vi "Do Something Else and Wait for Reply.vi"(6 "wait for reply (T)":bool=TRUE, 8 "error in (no error)":errorcluster, 9 "X":dbl, 10 "Do Something Else Message":string, 11 "Module ID":i32=-1) -> (0 "error out":errorcluster, 1 "timed out?":bool, 2 "Reply Payload":T1)   [LabVIEW 2018, in "CE14 eMIC module.lvlib"]
doc: "Send the Do Something Else request to the Module's Main.vi.\n_____\nBased on DQMH Project Template 6.0.0.91."
uses:
  CE14 eMIC module.lvlib
  Do Something Else and Wait (Reply Payload)--cluster.ctl
  Do Something Else and Wait for Reply Argument--cluster.ctl
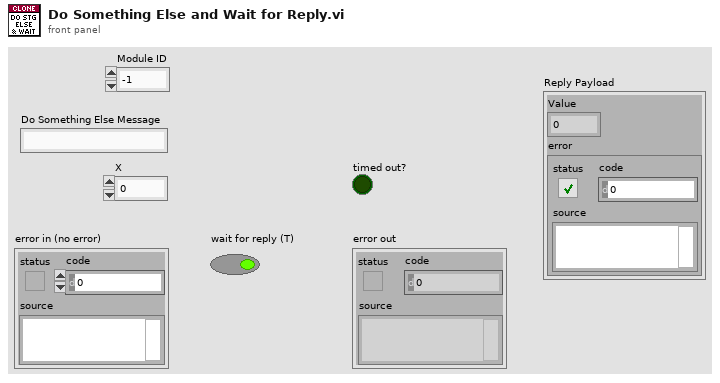
[diagram p1: front panel]
types:
  T1 = typedef "CE14 eMIC module.lvlib/Do Something Else and Wait (Reply Payload)--cluster.ctl" = cluster{"Value":dbl, "error":errorcluster}
  T2 = typedef "CE14 eMIC module.lvlib/Request Events--cluster.ctl" = cluster{"Stop Module":refnum<user-event>, "Do Something":refnum<user-event>, "Do Something Else":refnum<user-event>, "Do Something Else and Wait for Reply":refnum<user-event>, "Show Panel":refnum<user-event>, "Hide Panel":refnum<user-event>, "Show Diagram":refnum<user-event>, "Get Module Execution Status":refnum<user-event>, "Open&shakehand eMICs":refnum<user-event>, "Read ACV, ACI, PF, KW":refnum<user-event>, "CE14 Close":refnum<user-event>}
  T3 = typedef "CE14 eMIC module.lvlib/Do Something Else and Wait for Reply Argument--cluster.ctl" = cluster{"Module ID":i32, "Do Something Else Msg":string, "X":dbl, "Wait Notifier":refnum<notifier>, "wait for reply":bool}
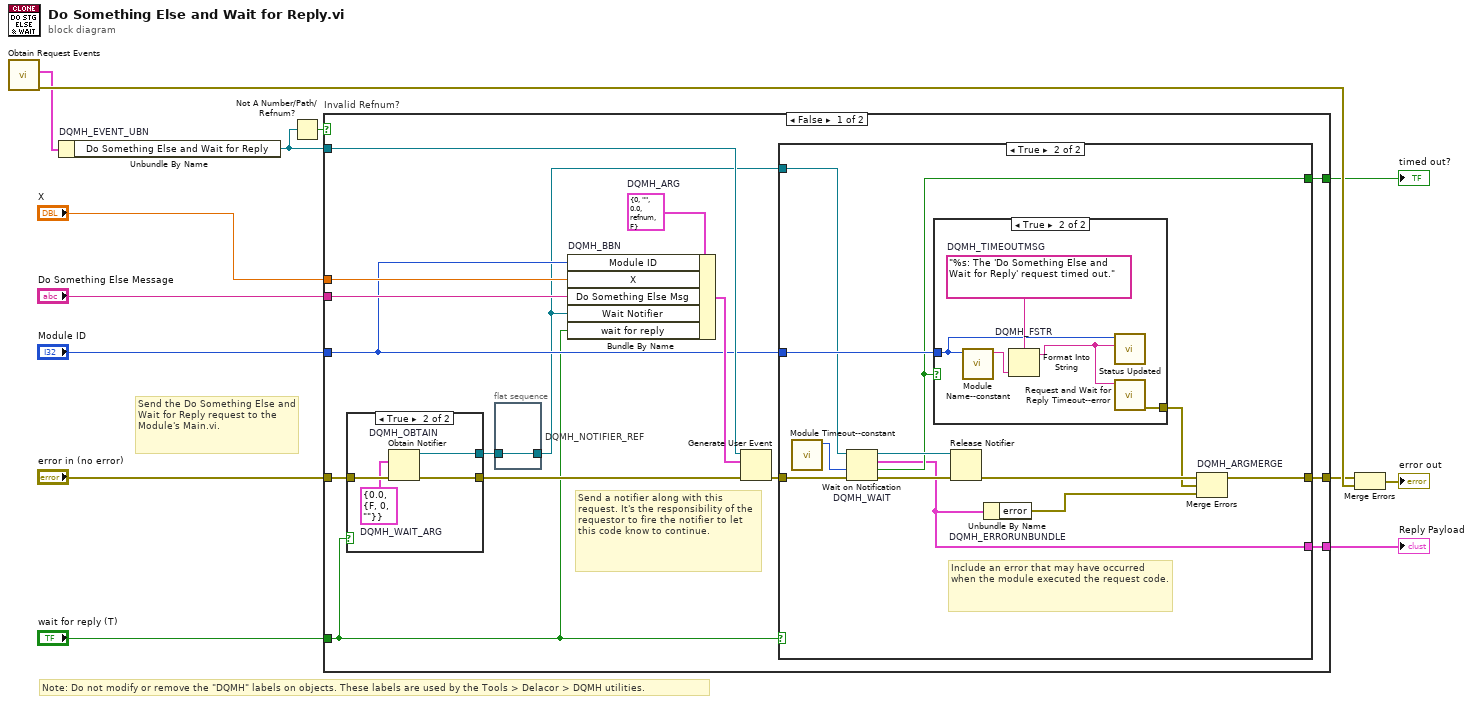
[diagram p0: block diagram]
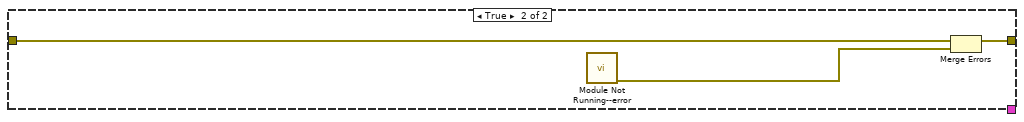
[diagram p5: hidden frame]
diagram:
  # "Note: Do not modify or remove the \"DQMH\" labels on objects. These labels are used by the Tools > Delacor > DQMH utilities."
  # "Send the Do Something Else and Wait for Reply request to the Module's Main.vi."
  n1 = call "Obtain Request Events.vi"() -> ("error out"=w12:errorcluster, "CE14 eMIC module Request Events"=w11:T2)  [unwired: 10 in]
  n2 = Unbundle By Name "DQMH_EVENT_UBN"(w11) -> ("Do Something Else and Wait for Reply"=w9:refnum<user-event>)
  n3 = Not A Number/Path/Refnum?(number/path/refnum=w9) -> (NaN/Path/Refnum?=w10:bool)
  n4 = case "Invalid Refnum?" shown="False" w10 {
    tunnel: [w18 w54] -> w5
    tunnel: "X" -> [w25 _]
    tunnel: "Do Something Else Message" -> [w24 _]
    tunnel: "error in (no error)" -> [w23 w53]
    tunnel: w9 -> [w22 _]
    tunnel: "Module ID" -> [w20 _]
    tunnel: [w19 _] -> w3
    tunnel: [w17 _] -> w2
    tunnel: "wait for reply (T)" -> [w14 _]
    frame False {
      w21 = T3 {"Module ID"=0, "Do Something Else Msg"="", "X"=0.0, "Wait Notifier"=refnum, "wait for reply"=FALSE}  # DQMH_ARG
      # "Send a notifier along with this request. It's the responsibility of the requestor to fire the notifier to let this code know to continue."
      n5 = case shown="True" w14 {
        tunnel: [w48 w52] -> w26
        tunnel: [_ w51] -> w16
        tunnel: w23 -> [w48 w50]
        frame False {
        }
        frame True {
          w49 = T1 {"Value"=0.0, "error"={"status"=FALSE, "code"=0, "source"=""}}  # DQMH_WAIT_ARG
          n6 = Obtain Notifier "DQMH_OBTAIN"(notification data type=w49, error in (no error)=w50) -> (notifier out=w51:refnum<notifier>, error out=w52:errorcluster)  [unwired: 2 in, 1 out]
        }
      }
      n7 = flat-sequence "DQMH_NOTIFIER_REF" {
        tunnel: w16 -> [w47]
        tunnel: [w47] -> w15
        frame #0 {
        }
      }
      n8 = Bundle By Name "DQMH_BBN"(cluster=w21, "Module ID"=w20, "X"=w25, "Do Something Else Msg"=w24, "Wait Notifier"=w15, "wait for reply"=w14) -> (w27:T3)
      n9 = Generate User Event(user event=w22, event data cluster=w27, error in=w26) -> (error out=w28:errorcluster)  [unwired: 1 in, 1 out]
      n10 = case shown="True" w14 {
        tunnel: w28 -> [w29 w40]
        tunnel: w20 -> [_ w36]
        tunnel: [_ w35] -> w19
        tunnel: [w29 w34] -> w18
        tunnel: [_ w33] -> w17
        tunnel: w15 -> [_ w32]
        frame False {
        }
        frame True {
          # "Include an error that may have occurred when the module executed the request code."
          n11 = call "Module Timeout--constant.vi"() -> ("Module Timeout"=w39:i32)  [unwired: 11 in]
          n12 = Wait on Notification "DQMH_WAIT"(notifier=w32, timeout in ms (-1)=w39, error in (no error)=w40) -> (notifier out=w38:refnum<notifier>, notification=w33:T1, timed out?=w35:bool, error out=w41:errorcluster)  [unwired: 1 in]
          n13 = case shown="True" w35 {
            tunnel: w36 -> [_ w44]
            tunnel: [_ w42] -> w30
            frame False {
            }
            frame True {
              w45 = "%s: The 'Do Something Else and Wait for Reply' request timed out."  # DQMH_TIMEOUTMSG
              n14 = call "Module Name--constant.vi"("Module ID"=w44) -> ("Module Name"=w46:string)  [unwired: 10 in]
              n15 = Format Into String "DQMH_FSTR"(format string=w45, w46) -> (resulting string=w43:string)  [unwired: 2 in, 1 out]
              n16 = call "Status Updated.vi"("Status"=w43, "Module ID"=w44) -> ()  [unwired: 9 in, 1 out]
              n17 = call "Request and Wait for Reply Timeout--error.vi"("Error Message"=w43) -> ("error out"=w42:errorcluster)  [unwired: 10 in]
            }
          }
          n18 = Release Notifier(notifier=w38, error in (no error)=w41) -> (error out=w37:errorcluster)  [unwired: 1 in, 2 out]
          n19 = Unbundle By Name "DQMH_ERRORUNBUNDLE"(w33) -> ("error"=w31:errorcluster)
          n20 = Merge Errors "DQMH_ARGMERGE"(w37, w30, w31) -> (w34:errorcluster)
        }
      }
    }
    frame True {
      n21 = call "Module Not Running--error.vi"() -> ("error out"=w55:errorcluster)  [unwired: 11 in]
      n22 = Merge Errors(w53, w55) -> (w54:errorcluster)
    }
  }
  "timed out?" <- w3
  "Reply Payload" <- w2
  n23 = Merge Errors(w5, w12) -> (→"error out":errorcluster)
